vi "Get End Tag.vi"(8 "error in (no error)":errorcluster, 11 "Data Item in":refnum<class "Data Item.lvclass">) -> (0 "error out":errorcluster, 2 "End Tag":string, 3 "Data Item out":refnum<class "Data Item.lvclass">)   [LabVIEW 2026, in "VILab.lvlib" / "Data Item.lvclass"]
uses:
  Data Item.lvclass
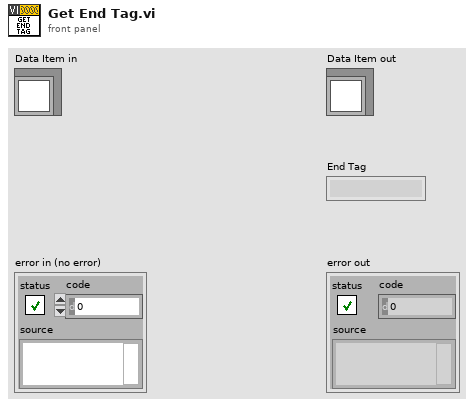
[diagram p1: front panel]
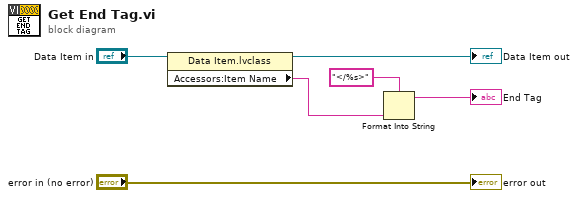
[diagram p0: block diagram]
diagram:
  n1 = property class="Data Item.lvclass"(reference="Data Item in") -> (reference out=→"Data Item out":refnum<class "Data Item.lvclass">, "Accessors:Item Name"=w1:string)  [unwired: 1 in, 1 out]
  n2 = Format Into String(format string="</%s>", w1) -> (resulting string=→"End Tag":string)  [unwired: 2 in, 1 out]
  "error out" <- "error in (no error)"
